vi "Handle Activate Menu On Tree Item.vi"(8 "error in (no error)":errorcluster, 9 "Coords":T1, 10 "MenuRef":refnum<k9>, 11 "Process Explorer View in":refnum<class "Process Explorer View.lvclass">) -> (0 "error out":errorcluster, 1 "Discard?":bool, 3 "Process Explorer View out":refnum<class "Process Explorer View.lvclass">)   [LabVIEW 2019, in "Process Explorer View.lvclass"]
doc: "<RequiredOverrideReason>Override to creae create custom right click menus in the file explorer.</RequiredOverrideReason>"
uses:
  <vilib>/gpm_packages/@cs/Car-wash/Source/Process Explorer View/Process Explorer View.lvclass
  C:/Program Files/National Instruments/LabVIEW 2019/vi.lib/gpm_packages/@cs/file-explorer-extension/Source/File Explorer/File Explorer/File Explorer.lvclass
  <vilib>/Utility/miscctls.llb/LVPoint32TypeDef.ctl
  <vilib>/gpm_packages/@cs/file-explorer-extension/Source/File Explorer/File Explorer/File Explorer.lvclass/File Explorer.ctl
  <vilib>/gpm_packages/@cs/file-explorer-extension/Source/File Explorer/File Explorer/File Explorer.lvclass
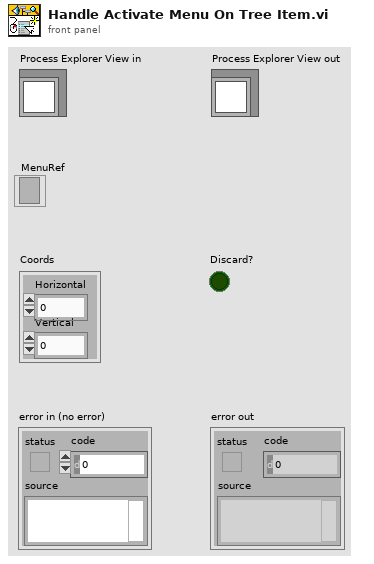
[diagram p1: front panel]
types:
  T1 = typedef "LVPoint32TypeDef.ctl" = cluster{"Horizontal":i32, "Vertical":i32}
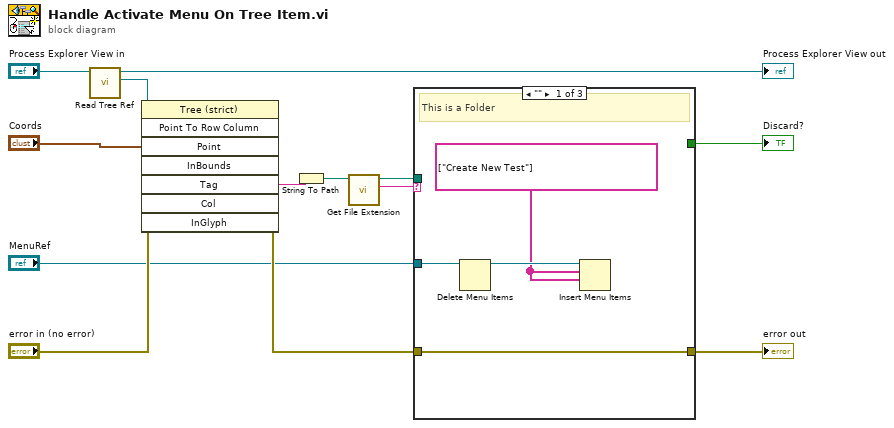
[diagram p0: block diagram]
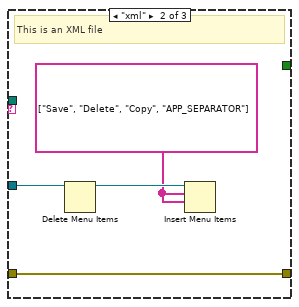
[diagram p2: hidden frame]
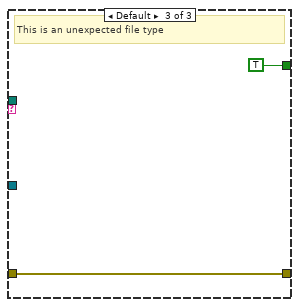
[diagram p3: hidden frame]
diagram:
  n1 = call <vilib>:"Read Tree Ref.vi"("File Explorer in"="Process Explorer View in") -> ("Tree Ref"=w13:refnum<vi>, "File Explorer out"=→"Process Explorer View out":refnum<class "Process Explorer View.lvclass">)  [unwired: 8 in, 1 out]
  n2 = invoke class="Tree (strict)" method="Point To Row Column"(reference=w13, error in="error in (no error)", "Point"="Coords") -> (error out=w9:errorcluster, "Tag"=w12:string)  [unwired: 5 in, 6 out]
  n3 = String To Path(string=w12) -> (path=w11:path)
  n4 = call <vilib>:"Get File Extension.vi"("file"=w11) -> ("lowercase file extension"=w10:string, "dup file"=w8:path)  [unwired: 6 in, 3 out]
  n5 = case shown="\"\"" w10 {
    tunnel: [_ _ TRUE] -> w1
    tunnel: [w17 w21 w22] -> w4
    tunnel: w9 -> [w17 w21 w22]
    tunnel: "MenuRef" -> [w16 w19 _]
    tunnel: w8 -> [_ _ _]
    frame "" {
      w14 = string[] ["Create New Test"] ("item names")
      # "This is a Folder"
      n6 = Delete Menu Items(9:w16) -> (3:w15:refnum<k9>)  [unwired: 3 in, 1 out]
      n7 = Insert Menu Items(7:w14, 8:w14, 9:w15) -> ()  [unwired: 3 in, 3 out]
    }
    frame "xml" {
      w18 = string[] ["Save", "Delete", "Copy", "APP_SEPARATOR"] ("item names")
      # "This is an XML file"
      n8 = Delete Menu Items(9:w19) -> (3:w20:refnum<k9>)  [unwired: 3 in, 1 out]
      n9 = Insert Menu Items(7:w18, 8:w18, 9:w20) -> ()  [unwired: 3 in, 3 out]
    }
    frame Default {
      # "This is an unexpected file type"
    }
  }
  "error out" <- w4
  "Discard?" <- w1
